vi "Modes_Open Area.vi"(11 "Mode":u16(ring) items=["Drive into AUTO Zone"]) -> ()   [LabVIEW 2014]
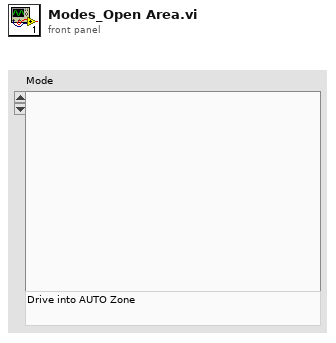
[diagram p1: front panel]
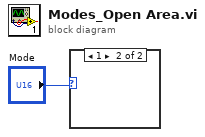
[diagram p0: block diagram]
diagram:
  n1 = case shown="1" "Mode" {
    frame 0, Default {
    }
    frame 1 {
    }
  }
